vi "DAQmx_String to Input Term Config Ring.vi"(8 "error in (no error)":errorcluster, 11 "Input TermCfg Str":string) -> (0 "error out":errorcluster, 3 "input terminal configuration":i32(ring)=10106 items=["default"=-1, "RSE"=10083, "NRSE"=10078, "Differential"=10106, "Pseudodifferential"=12529])   [LabVIEW 2012]
doc: "Converts a string to the \"input terminal configuration\" ring type."
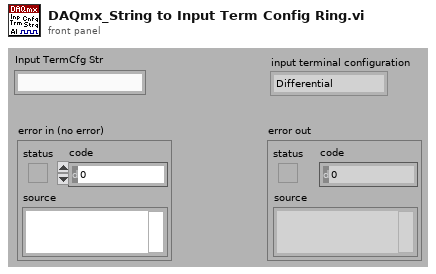
[diagram p1: front panel]
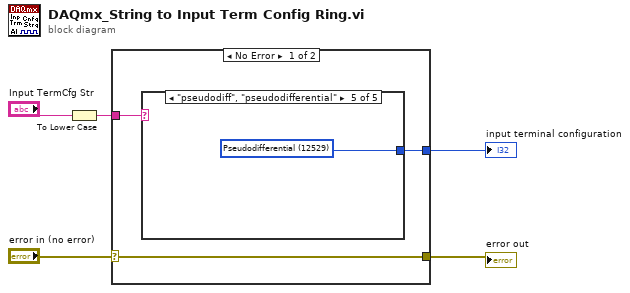
[diagram p0: block diagram]
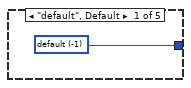
[diagram p2: hidden frame]
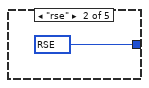
[diagram p3: hidden frame]
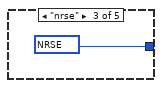
[diagram p4: hidden frame]
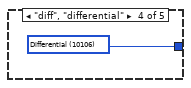
[diagram p5: hidden frame]
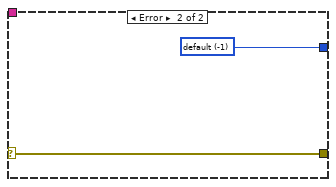
[diagram p6: hidden frame]
diagram:
  n1 = To Lower Case(string="Input TermCfg Str") -> (all lower case string=w1:string)
  n2 = case shown="No Error" "error in (no error)" {
    selector: "error in (no error)" -> [w6 w15]
    tunnel: w1 -> [w8 _]
    tunnel: [w7 w14] -> w4
    tunnel: [w6 w15] -> w2
    frame No Error {
      n3 = case shown="\"pseudodiff\", \"pseudodifferential\"" w8 {
        tunnel: [w9 w10 w11 w12 w13] -> w7
        frame "default", Default {
          w9 = -1 items=["default"=-1, "RSE"=10083, "NRSE"=10078, "Differential"=10106, "Pseudodifferential"=12529] ("input terminal configuration")
        }
        frame "rse" {
          w10 = 10083 items=["default"=-1, "RSE"=10083, "NRSE"=10078, "Differential"=10106, "Pseudodifferential"=12529] ("input terminal configuration")
        }
        frame "nrse" {
          w11 = 10078 items=["default"=-1, "RSE"=10083, "NRSE"=10078, "Differential"=10106, "Pseudodifferential"=12529] ("input terminal configuration")
        }
        frame "diff", "differential" {
          w12 = 10106 items=["default"=-1, "RSE"=10083, "NRSE"=10078, "Differential"=10106, "Pseudodifferential"=12529] ("input terminal configuration")
        }
        frame "pseudodiff", "pseudodifferential" {
          w13 = 12529 items=["default"=-1, "RSE"=10083, "NRSE"=10078, "Differential"=10106, "Pseudodifferential"=12529] ("input terminal configuration")
        }
      }
    }
    frame Error {
      w14 = -1 items=["default"=-1, "RSE"=10083, "NRSE"=10078, "Differential"=10106, "Pseudodifferential"=12529] ("input terminal configuration")
    }
  }
  "input terminal configuration" <- w4
  "error out" <- w2
